vi "4_Virtual_Channels.vi"() -> ()   [LabVIEW 2015]
uses:
  C:/Users/MX-Microscope/Documents/LabVIEW Data/lvoop_campus_2018/Detector_Class/Swabian/time_tagger_vis/TTCSharp32.dll
  TTCSharp32.dll
panel:
  out "getData":dbl[](array[numeric])
  # "Here, we have used a coincidence window that coincides just with the propagation delay\nbetween ch0 and ch1. Due to jitter, approximately half of the coincidence counts\nfall outside of this coincidence range. Therefore the coincidence countrate is\napproximately half of the original count rate."
  # "channel 0"
  # "in counts / s"
  # "channel 0 and channel 1"
  # "coincidences"
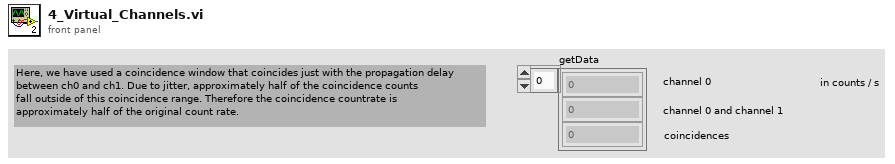
[diagram p1: front panel]
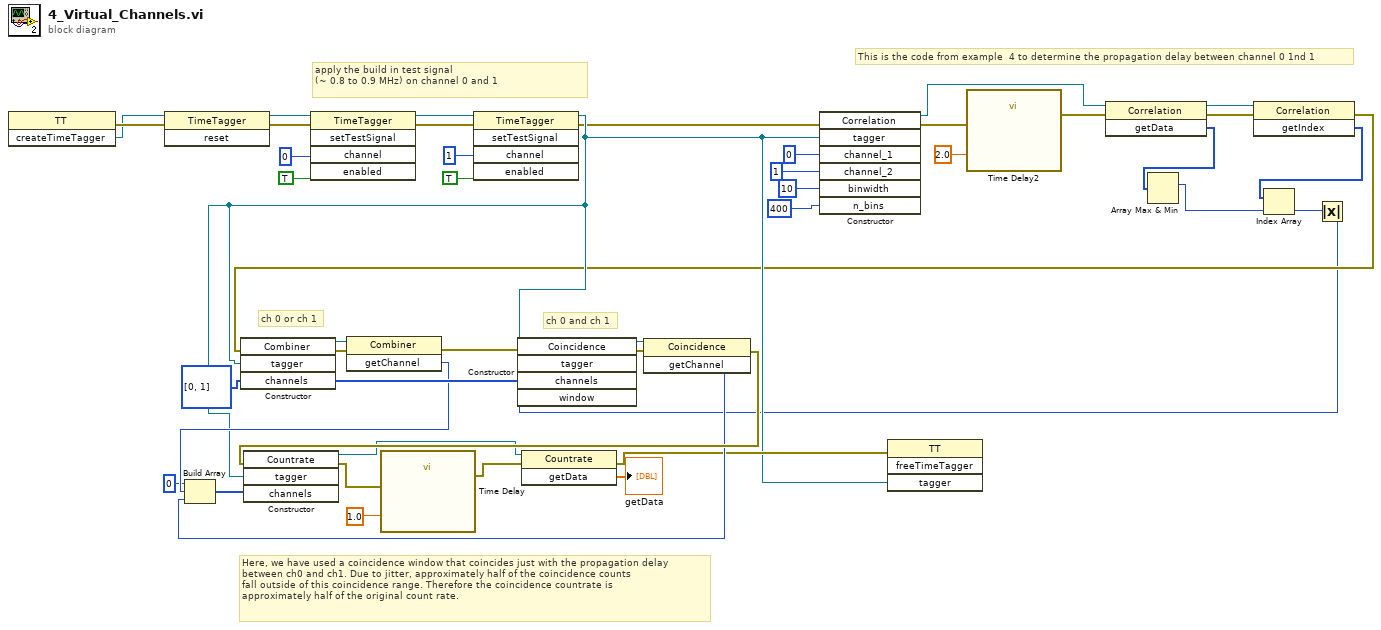
[diagram p0: block diagram]
diagram:
  # "ch 0 and ch 1"
  # "ch 0 or ch 1"
  # "This is the code from example  4 to determine the propagation delay between channel 0 1nd 1"
  # "Here, we have used a coincidence window that coincides just with the propagation delay\nbetween ch0 and ch1. Due to jitter, approximately half of the coincidence counts\nfall outside of this coincidence range. Therefore the coincidence countrate is\napproximately half of the original count rate."
  # "apply the build in test signal\n(~ 0.8 to 0.9 MHz) on channel 0 and 1"
  n1 = invoke class="TT" method="createTimeTagger"() -> (error out=w42:errorcluster, "createTimeTagger"=w41:refnum<k24>)  [unwired: 3 in, 1 out]
  n2 = invoke class="TimeTagger" method="reset"(reference=w41, error in=w42) -> (reference out=w37:refnum<k24>, error out=w38:errorcluster)  [unwired: 1 in, 1 out]
  n3 = invoke class="TimeTagger" method="setTestSignal"(reference=w37, error in=w38, "channel"=u32 0, "enabled"=TRUE) -> (reference out=w39:refnum<k24>, error out=w40:errorcluster)  [unwired: 1 in, 3 out]
  n4 = invoke class="TimeTagger" method="setTestSignal"(reference=w39, error in=w40, "channel"=u32 1, "enabled"=TRUE) -> (reference out=w8:refnum<k24>, error out=w7:errorcluster)  [unwired: 1 in, 3 out]
  n5 = constructor class="Correlation"(error in=w7, "tagger"=w8, "channel_1"=u32 0, "channel_2"=u32 1, "binwidth"=i64 10, "n_bins"=400) -> (reference out=w9:refnum<k24>, error out=w10:errorcluster)  [unwired: 2 in, 6 out]
  n6 = call "Time Delay2"("error in (no error)"=w10, "Delay Time (s)"=2.0) -> ("error out"=w11:errorcluster)  [unwired: 9 in]
  n7 = invoke class="Correlation" method="getData"(reference=w9, error in=w11) -> (reference out=w18:refnum<k24>, error out=w17:errorcluster, "getData"=w6:i32[])  [unwired: 1 in]
  n8 = Array Max & Min(array=w6) -> (max index (indices)=w5:i32)  [unwired: 3 out]
  n9 = invoke class="Correlation" method="getIndex"(reference=w18, error in=w17) -> (error out=w3:errorcluster, "getIndex"=w4:i64[])  [unwired: 1 in, 1 out]
  n10 = constructor class="Combiner"(error in=w3, "tagger"=w8, "channels"=u32[] [0, 1]) -> (reference out=w33:refnum<k24>, error out=w32:errorcluster, "channels"=w34:u32[])  [unwired: 2 in, 2 out]
  n11 = invoke class="Combiner" method="getChannel"(reference=w33, error in=w32) -> (error out=w31:errorcluster, "getChannel"=w27:u32)  [unwired: 1 in, 1 out]
  n12 = Index Array(array=w4, index=w5) -> (element=w2:i64)
  n13 = Absolute Value(x=w2) -> (abs(x)=w1:i64)
  n14 = constructor class="Coincidence"(error in=w31, "tagger"=w8, "channels"=w34, "window"=w1) -> (reference out=w30:refnum<k24>, error out=w29:errorcluster)  [unwired: 2 in, 4 out]
  n15 = invoke class="Coincidence" method="getChannel"(reference=w30, error in=w29) -> (error out=w28:errorcluster, "getChannel"=w26:u32)  [unwired: 1 in, 1 out]
  n16 = Build Array(u32 0 ("element"), w27, w26) -> (w25:u32[])
  n17 = constructor class="Countrate"(error in=w28, "tagger"=w8, "channels"=w25) -> (reference out=w21:refnum<k24>, error out=w23:errorcluster)  [unwired: 2 in, 3 out]
  n18 = call "Time Delay"("error in (no error)"=w23, "Delay Time (s)"=1.0) -> ("error out"=w22:errorcluster)  [unwired: 9 in]
  n19 = invoke class="Countrate" method="getData"(reference=w21, error in=w22) -> (error out=w19:errorcluster, "getData"=→"getData":dbl[])  [unwired: 1 in, 1 out]
  n20 = invoke class="TT" method="freeTimeTagger"(error in=w19, "tagger"=w8) -> ()  [unwired: 2 in, 4 out]
